vi "sv_Convert String to Value (Specific Datatype).vi"(7 "specific data type string":string) -> (8 "specific data type value":T1 items=["unknown"=0, "general"=1, "stress"=2, "strain"=3, "temperature"=5, "heat flux"=6, "displacement"=8, "reaction force"=9, "velocity"=11, "acceleration"=12, "excitation force"=13, "pressure"=15, "mass"=16, "time"=17, "frequency"=18, "rpm"=19, "order"=20, "sound pressure"=21, "sound intensity"=22, "sound power"=23])   [LabVIEW 2017, in "SoundVib_UFF58.lvlib"]
uses:
  <vilib>/addons/Sound and Vibration/svt_UFF58/SoundVib_UFF58.lvlib
  <vilib>/addons/Sound and Vibration/svt_UFF58/subVIs/sv_UFF58 Specific Datatype.ctl
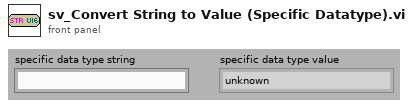
[diagram p1: front panel]
types:
  T1 = typedef "SoundVib_UFF58.lvlib/sv_UFF58 Specific Datatype.ctl" = u16
  T2 = typedef "SoundVib_UFF58.lvlib/sv_UFF58 Specific Datatype Array.ctl" = string[]
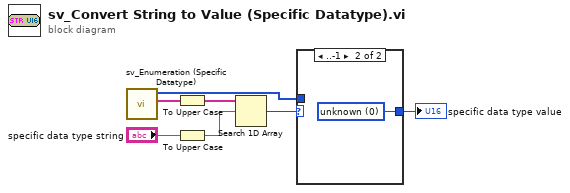
[diagram p0: block diagram]
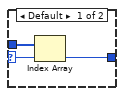
[diagram p2: hidden frame]
diagram:
  n1 = call <vilib>:"sv_Enumeration (Specific Datatype).vi"() -> ("specific datatype strings"=w2:T2, "specific datatype U16 values"=w1:u16[])  [unwired: 10 in]
  n2 = To Upper Case(1:w2) -> (0:w6:T2)
  n3 = To Upper Case(1:"specific data type string") -> (0:w5:string)
  n4 = Search 1D Array(1D array=w6, element=w5) -> (index of element=w4:i32)  [unwired: 1 in]
  n5 = case shown="..-1" w4 {
    selector: w4 -> [w10 _]
    tunnel: w1 -> [w9 _]
    tunnel: [w8 w11] -> w3
    frame Default {
      n6 = Index Array(array=w9, index=w10) -> (element=w8:u16)
    }
    frame ..-1 {
      w11 = T1 0 items=["unknown"=0, "general"=1, "stress"=2, "strain"=3, "temperature"=5, "heat flux"=6, "displacement"=8, "reaction force"=9, "velocity"=11, "acceleration"=12, "excitation force"=13, "pressure"=15, "mass"=16, "time"=17, "frequency"=18, "rpm"=19, "order"=20, "sound pressure"=21, "sound intensity"=22, "sound power"=23] ("specific data type")
    }
  }
  "specific data type value" <- w3
